vi "Type Testing.vi"(10 "Cluster":T4) -> (0 "Type 2":T1, 1 "VI Server Generic Type":T2, 2 "Reference Type":T3, 3 "Type":T1)   [LabVIEW 2018]
uses:
  <vilib>/Utility/Data Type/Type Definitions/Data Type.ctl
  <vilib>/Utility/Data Type/Type Definitions/Refnum Type.ctl
  <vilib>/Utility/Data Type/Type Definitions/VI Server Generic Type.ctl
  <vilib>/Utility/Data Type/NI_Data Type.lvlib
panel:
  out "Cluster Elements":variant[](array[variant])
  out "Strict Type":variant
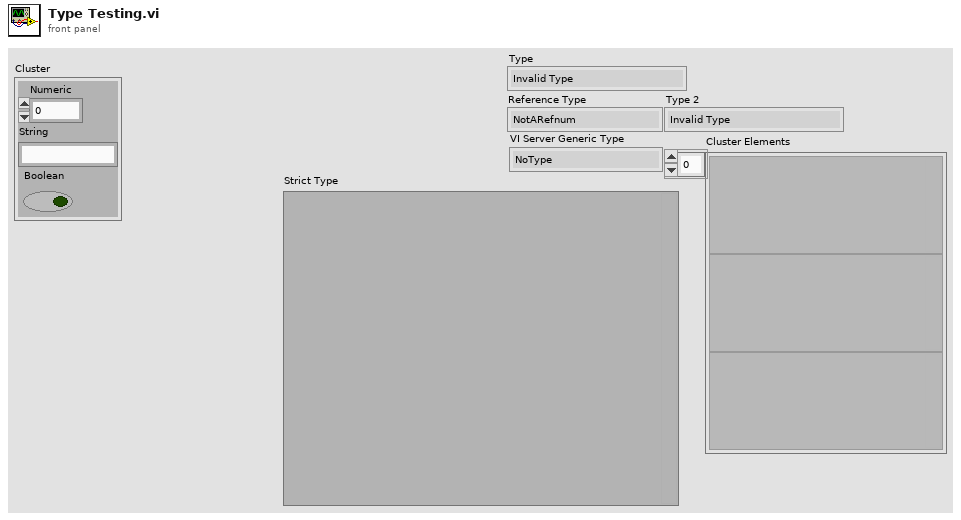
[diagram p1: front panel]
types:
  T1 = typedef "NI_Data Type.lvlib/Data Type.ctl" = enum8{"Invalid Type", "Void", "I8", "I16", "I32", "I64", "U8", "U16", "U32", "U64", "Single Float", "Double Float", "Extended Float", "Single Complex", "Double Complex", "Extended Complex", "Enum U8", "Enum U16", "Enum U32", "Enum U64", "Single Float With Unit", "Double Float With Unit", "Extended Float With Unit", "Single Complex with Unit", "Double Complex with Unit", "Extended Complex with Unit", "Boolean", "String", "Path", "Picture", "Tag", "Array", "Cluster", "Variant", "LV Variant", "Waveform", "Timestamp", "Digital Waveform", "Digital Data", "ExpressData", "Refnum", "External Data", "VI", "Poly VI", "LabVIEW Class Instance", "Fixed Point"}
  T2 = typedef "NI_Data Type.lvlib/VI Server Generic Type.ctl" = enum16{"NoType", "\tkLVObjApp=0x1", "\tkLVObjVI", "\tkLVObjGeneric", "\tkLVObjDecoration", "\tkLVObjText", "\tkLVObjControl", "\tkLVObjColorBox", "\tkLVObjBoolean", "\tkLVObjRefNum", "\tkLVObjVariant", "\tkLVObjPath", "\tkLVObjListBox", "\tkLVObjTable", "\tkLVObjArray", "\tkLVObjPicture", "\tkLVObjOleContainer", "\tkLVObjNumeric", "\tkLVObjDigital", "\tkLVObjNamedNumeric", "\tkLVObjColorRamp", "\tkLVObjSlide", "\tkLVObjGraphOrChart", "\tkLVObjWaveformChart", "\tkLVObjWaveformGraph", "\tkLVObjIntensityChart", "\tkLVObjIntensityGraph", "\tkLVObjString", "\tkLVObjIOName", "\tkLVObjComboBox", "\tkLVObjCluster", "\tkLVObjPanel", "\tkLVObjKnob", "\tkLVObjNumWithScale", "\tkLVObjRing", "\tkLVObjEnum", "\tkLVObjGObject", "\tkLVObjPlot", "\tkLVObjCursor", "\tkLVObjNumericText", "\tkLVObjScale", "\tkLVObjColorScale", "\tkLVObjGraphScale", "\tkLVObjColorGraphScale", "\tkLVObjTypedRefNum", "\tkLVObjOldKnobScale", "\tkLVObjMCListbox", "\tkLVObjMeasureData", "\tkLVObjDSCTag", "\tkLVObjDAQName", "\tkLVObjVISAName", "\tkLVObjIVIName", "\tkLVObjSlideScale", "\tkLVObjTabControl", "\tkLVObjPage", "\tkLVObjTabArrayTabControl", "\tkLVObjConPane", "\tkLVObjDAQMXName", "\tkLVObjVIRefNum", "\tkLVObjLVObjRefNum", "\tkLVObjAbsTime", "\tkLVObjDigitalTable", "\tkLVObjUnused", "\tkLVObjUnused2", "\tkLVObjSCLControl", "\tkLVObjSubPanel", "\tkLVObjTreeControl", "\tkLVObjGenClassTagRef", "\tkLVObjGenClassRef", "\tkLVObjRotaryColorScale", "\tkLVObjPlugInDDOControl", "\tkLVObjPlugInDDOClassHolder", "\tkLVObjRadClusControl", "\tkLVObjProject", "\tkLVObjProjectItem", "\tkLVObjPane", "\tkLVObjSplitterBar", "\tkLVObjProjectBuildItem", "\tkLVObjPixmap", "\tkLVObjFacadeVI", "\tkLVObjLibrary", "\tkLVObjVariable", "\tkLVObjPropertyBag", "\tkLVObjXYGraph", "\tkLVObjScene", "\tkLVObjUDClassLibrary", "\tkLVObjUDClassClone", "\tkLVObjMethodVI", "\tkLVObjXCtlLibrary", "\tkLVObjXNodeLibrary", "\tkLVObjScroll", "\tkLVObjLVTarget", "\tkLVObjMixedGraph", "\tkLVObjProvider", "\tkLVObjCopyOperation", "\tkLVObjTargetItem", "\tkLVObjProjectItemType", "\tkLVObjCopyItem", "\tkLVObjCopyConflict", "\tkLVObjCopyExpert", "\tkLVObjSceneGraphDisp", "\tkLVObjPolyVI", "\tkLVObjLVClassDDO", "kLVObjDiagram=0x4000", "\tkLVObjTerminal", "\tkLVObjConstant", "\tkLVObjPathConstant", "\tkLVObjArrayConstant", "\tkLVObjNumericConstant", "\tkLVObjDigitalNumConstant", "\tkLVObjNamedNumericConstant", "\tkLVObjStringConstant", "\tkLVObjClusterConstant", "\tkLVObjFixedConstant", "\tkLVObjControlTerminal", "\tkLVObjFormulaParameter", "\tkLVObjGlobal", "\tkLVObjLocal", "\tkLVObjRightShiftRegister", "\tkLVObjFunction", "\tkLVObjSubVI", "\tkLVObjCallByRef", "\tkLVObjUnitCast", "\tkLVObjStructure", "\tkLVObjLoop", "\tkLVObjMultiframeStructure", "\tkLVObjSequence", "\tkLVObjCaseSelector", "\tkLVObjFormula", "\tkLVObjGrowableFunction", "\tkLVObjBuildClusterArray", "\tkLVObjCompoundArithmetic", "\tkLVObjIndexArray", "\tkLVObjBuildArray", "\tkLVObjNamedBundler", "\tkLVObjCIN", "\tkLVObjCallLibrary", "\tkLVObjObjectFunction", "\tkLVObjProperty", "\tkLVObjInvoke", "\tkLVObjNode", "\tkLVObjBooleanConstant", "\tkLVObjBlockDiagram", "\tkLVObjRingConstant", "\tkLVObjEnumConstant", "\tkLVObjTunnel", "\tkLVObjLoopTunnel", "\tkLVObjSequenceLocal", "\tkLVObjComparison", "\tkLVObjReadWriteFile", "\tkLVObjTypeCast", "\tkLVObjFlattenUnflattenString", "\tkLVObjGPIBReadWrite", "\tkLVObjForLoop", "\tkLVObjWhileLoop", "\tkLVObjScriptNode", "\tkLVObjArrayToCluster", "\tkLVObjFormatScanString", "\tkLVObjWire", "\tkLVObjProbe", "\tkLVObjInnerTerminal", "\tkLVObjLeftShiftRegister", "\tkLVObjPolySubVI", "\tkLVObjPropItem", "\tkLVObjIONameConstant", "\tkLVObjDSCTagConstant", "\tkLVObjDAQNameConstant", "\tkLVObjVISANameConstant", "\tkLVObjIVINameConstant", "\tkLVObjColorBoxConstant", "\tkLVObjControlRefConstant", "\tkLVObjClassSpecifierConstant", "\tkLVObjConfNode", "\tkLVObjMasterWizard", "\tkLVObjStateDiagWizard", "\tkLVObjOuterTerminal", "\tkLVObjDAQMXNameConstant", "\tkLVObjEventStructure", "\tkLVObjFlatSequence", "\tkLVObjGenClassTagRefConstant", "\tkLVObjAbsTimeConstant", "\tkLVObjExternalNode", "\tkLVObjSubWizard", "\tkLVObjScriptNodeParameter", "\tkLVObjStatVIRef", "\tkLVObjComboBoxConstant", "\tkLVObjTimedLoop", "\tkLVObjGenClassDeepCopy", "\tkLVObjGenClassTagFlat", "\tkLVObjGenClassTagFlatRefConstant", "\tkLVObjGenClassFlat", "\tkLVObjSimDiagram", "\tkLVObjCompDiagram", "\tkLVObjSimNode", "\tkLVObjSimDCO", "\tkLVObjBundler", "\tkLVObjUnbundler", "\tkLVObjNamedUnbundler", "\tkLVObjFlatSeqFrame", "\tkLVObjFlatSeqInTun", "\tkLVObjFlatSeqOutTun", "\tkLVObjRefNumConst", "\tkLVObjFlattenString", "\tkLVObjPolySelector", "\tkLVObjXNode", "\tkLVObjSelectorTunnel", "\tkLVObjCommentNode", "\tkLVObjSdfDiagram", "\tkLVObjSDFCompDiagram", "\tkLVObjSdfNode", "\tkLVObjSdfDCO", "\tkLVObjFileDialog", "\tkLVObjTLDCO", "\tkLVObjTimeSeqFrame", "\tkLVObjTimeFlatSequence", "\tkLVObjTimedSequence", "\tkLVObjXDataNode", "\tkLVObjCodeWizard", "\tkLVObjMathScriptNode", "\tkLVObjMathScriptNodeParameter", "\tkLVObjLVClassBDConst"}
  T3 = typedef "NI_Data Type.lvlib/Refnum Type.ctl" = enum16{"NotARefnum", "UnknownRefnum", "Generic", "Datalog", "ByteStream", "Device", "Occurence", "TCPNetConnection", "Auto", "Menu", "Imaq", "Hardware", "DataSocket", "Visa", "IVI", "UDPNetConnection", "Notifier", "Queue", "Irda", "EventReg", "DotNet", "UserEvent", "Callback", "UNUSED_EMPTY_POSITION", "BlueToothNetConnection", "LVObjApp", "LVObjVI", "LVObjUnknown", "GenericClass", "UserDefinedRefnumTag", "DataValue", "RT FIFO", "TDMS File", "PythonSessionRefnum"}
  T4 = cluster{"Numeric":i32, "String":string, "Boolean":bool}
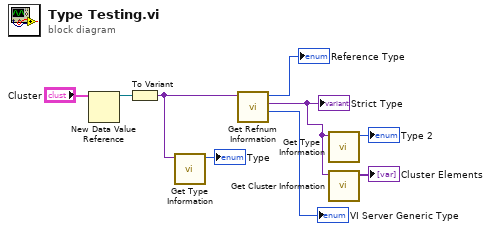
[diagram p0: block diagram]
diagram:
  n1 = New Data Value Reference(data value="Cluster") -> (data value reference=w8:refnum<data-value>)  [unwired: 1 in, 1 out]
  n2 = To Variant(anything=w8) -> (Variant=w6:variant)
  n3 = call <vilib>:"Get Type Information.vi"("Variant"=w6) -> ("Type"=→"Type":T1)  [unwired: 6 in, 4 out]
  n4 = call <vilib>:"Get Refnum Information.vi"("Variant"=w6) -> ("VI Server Generic Type"=→"VI Server Generic Type":T2, "Strict Type"=w2:variant, "Reference Type"=→"Reference Type":T3)  [unwired: 7 in, 1 out]
  "Strict Type" <- w2
  n5 = call <vilib>:"Get Type Information.vi"("Variant"=w2) -> ("Type"=→"Type 2":T1)  [unwired: 6 in, 4 out]
  n6 = call <vilib>:"Get Cluster Information.vi"("Variant"=w2) -> ("Cluster Elements"=→"Cluster Elements":variant[])  [unwired: 9 in, 1 out]
